vi "Cash_check.vi"(8 "error in (no error)":errorcluster, 9 "Empty":bool, 10 "cash":dbl, 11 "input":string) -> (0 "error out":errorcluster, 2 "new cash":ext, 3 "ATM window":string)   [LabVIEW 2025]
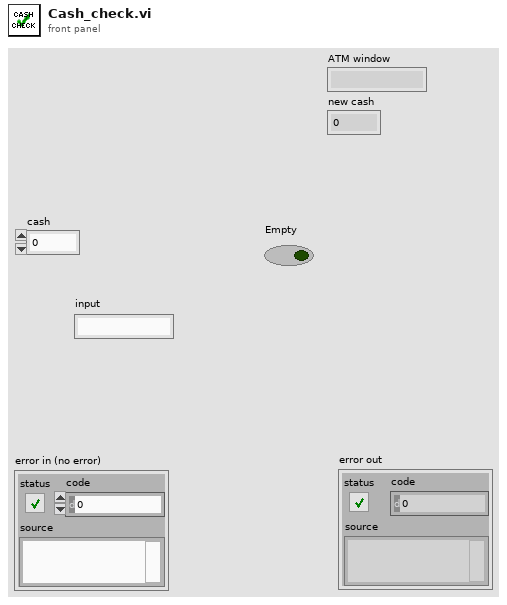
[diagram p1: front panel]
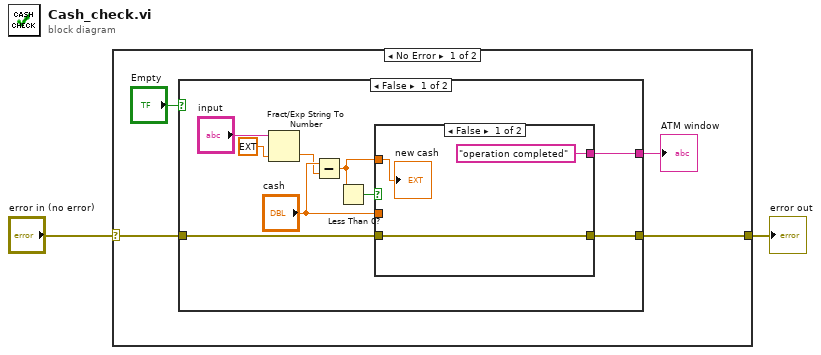
[diagram p0: block diagram]
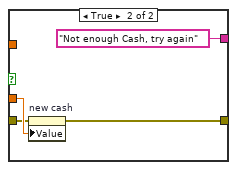
[diagram p2: hidden frame]
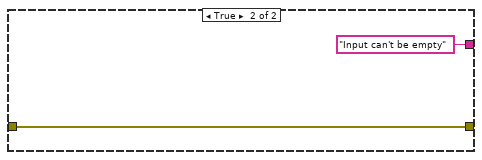
[diagram p3: hidden frame]
diagram:
  n1 = case shown="No Error" "error in (no error)" {
    selector: "error in (no error)" -> [w4 w25]
    tunnel: [w3 w25] -> w1
    frame No Error {
      n2 = case shown="False" "Empty" {
        tunnel: [w12 "Input can't be empty"] -> w5
        tunnel: w4 -> [w10 w23]
        tunnel: [w9 w23] -> w3
        frame False {
          n3 = Fract/Exp String To Number(string="input", default (0 dbl)=ext 0.0 ("default (0 DBL)")) -> (number=w7:ext)  [unwired: 2 in, 1 out]
          n4 = Subtract(x="cash", y=w7) -> (x-y=w11:ext)
          n5 = Less Than 0?(x=w11) -> (x < 0?=w13:bool)
          n6 = case shown="False" w13 {
            tunnel: ["operation completed" ("input") "Not enough Cash, try again" ("input")] -> w12
            tunnel: w11 -> [w17 _]
            tunnel: "cash" -> [_ w21]
            tunnel: w10 -> [w16 w20]
            tunnel: [w16 w19] -> w9
            frame False {
              "new cash" <- w17
            }
            frame True {
              n7 = property on="new cash" class="DigNum (strict)"(error in=w20, "Value"=w21) -> (error out=w19:errorcluster)  [unwired: 1 in, 1 out]
            }
          }
        }
        frame True {
        }
      }
      "ATM window" <- w5
    }
    frame Error {
    }
  }
  "error out" <- w1
